vi "Patrick Builder.vi"() -> ()   [LabVIEW 2019, in "VIPM.lvclass"]
uses:
  VIPM.lvclass
  Typedefs/File Type--enum.ctl
  <vilib>/Utility/sysdir.llb/System Directory Type.ctl
  <vilib>/Utility/file.llb/Read Delimited Spreadsheet (string).vi
  <vilib>/Utility/file.llb/Write Delimited Spreadsheet (string).vi
  <vilib>/JKI/VIPM API/VIPM API_vipm_api.lvlib
panel:
  in  "Mode":T1
  in  "Create File List":bool
  out "Package Builder":string
  in  "Clear Notes":bool
  in  "Release Notes":string
  in  "Append Notes":bool
  in  "ALL":bool
  in  "Patch +1":bool
  out "Selected File List":string
  in  "Publish":bool
  in  "Open List":bool
  in  "Build":bool
  in  "Preview":bool
  out "Status":string
  in  "File List":i32(listbox)
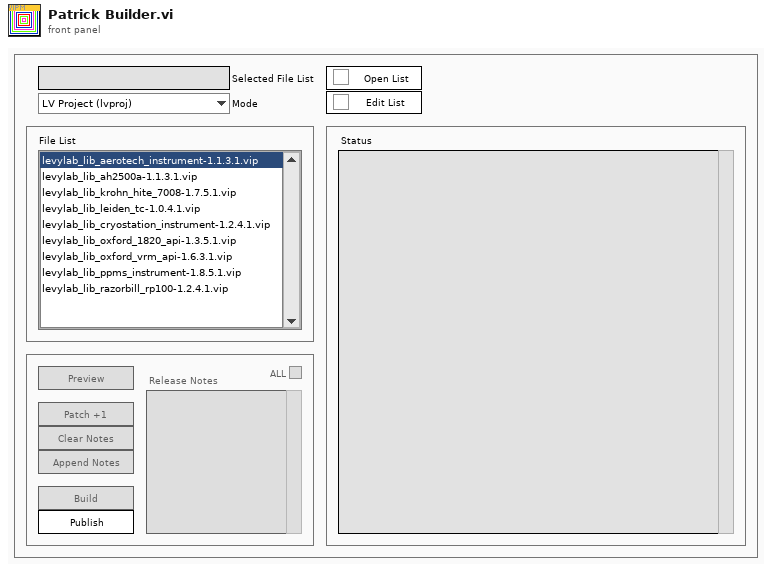
[diagram p1: front panel]
types:
  T1 = typedef "VIPM.lvclass/File Type--enum.ctl" = enum16{"LV Project (lvproj)", "Build Spec (vipb)", "Package (vip)"}
  T2 = enum32{"Invalid", "Standard", "Closed", "Hidden", "Minimized", "Maximized"}
  T3 = enum32{"invalid app kind", "Development System", "Run Time System", "Student Edition", "Embedded LabVIEW", "Evaluation", "Custom"}
  T4 = enum8{"Enabled", "Disabled", "Disabled and Grayed Out"}
  T5 = cluster{"Core":cluster{"Current VI Reference":refnum<vi>, "Close Panel on Exit?":bool}, "lvproj paths":path[], "vipb paths":path[], "vip paths":path[], "selected path":path, "config path":path, "Mode":T1}
  T6 = typedef "System Directory Type.ctl" = i32
  T7 = cluster{"Current VI Reference":refnum<vi>, "Close Panel on Exit?":bool}
  T8 = typedef "VIPM API_vipm_api.lvlib/VI Package Build Spec Data Cluster_vipm_api.ctl" = cluster{"Package Version":T9, "Product Name":string, "Company Name":string, "Author Name (Person or Company)":string, "Product Homepage (URL)":string, "Legal Copyright":string, "License Agreement Name":string, "Product Description Summary":string, "Product Description":string, "Release Notes - Change Log":string}
  T9 = typedef "VIPM API_vipm_api.lvlib/Version Info Cluster_vipm_api.ctl" = cluster{"major":u32, "minor":u32, "patch":u32, "build":u32}
  T10 = typedef "VIPM API_vipm_api.lvlib/Repository Info Cluster_vipm_api.ctl" = cluster{"Repository Name":string, "Repository Folder Location":path}
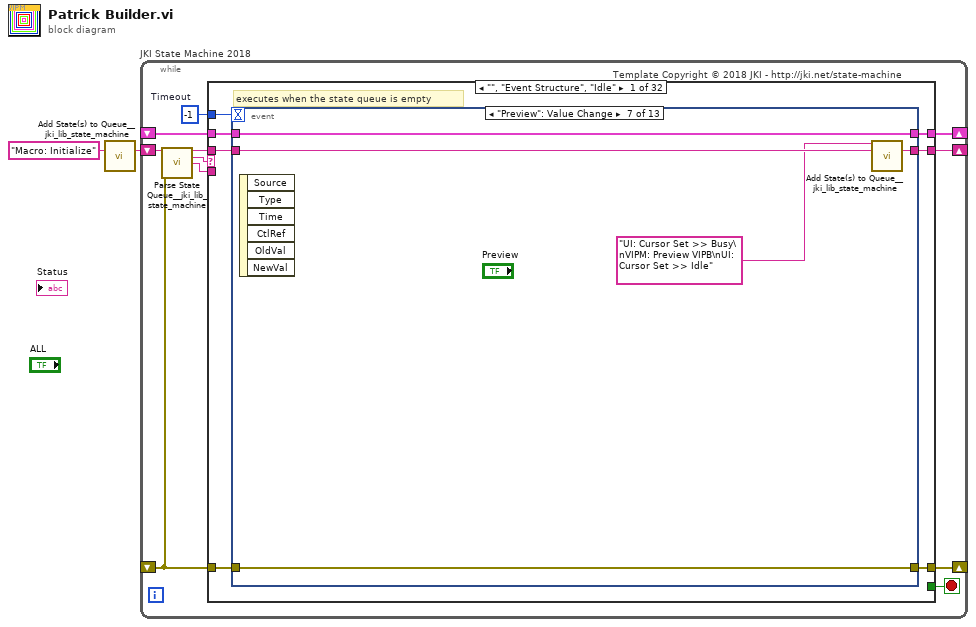
[diagram p0: block diagram]
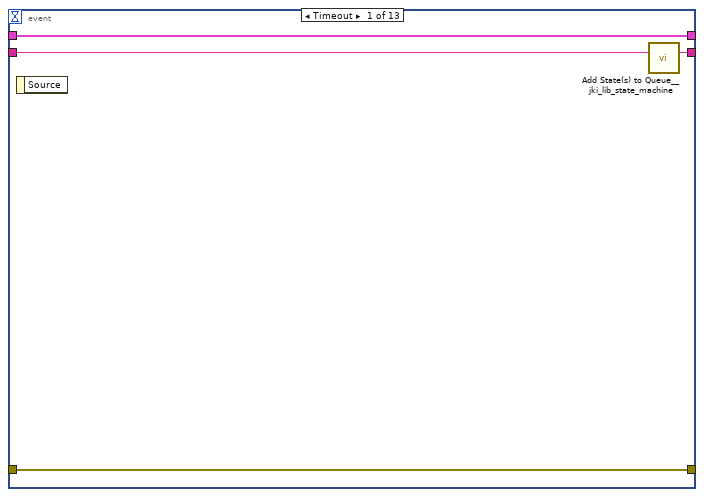
[diagram p2: hidden frame]
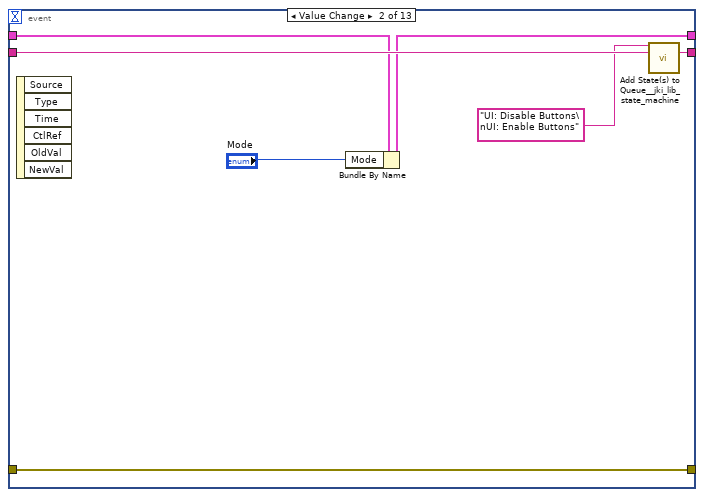
[diagram p3: hidden frame]
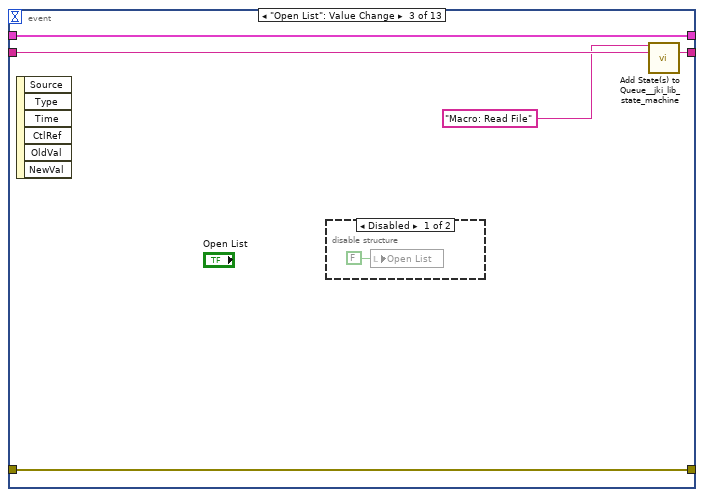
[diagram p4: hidden frame]
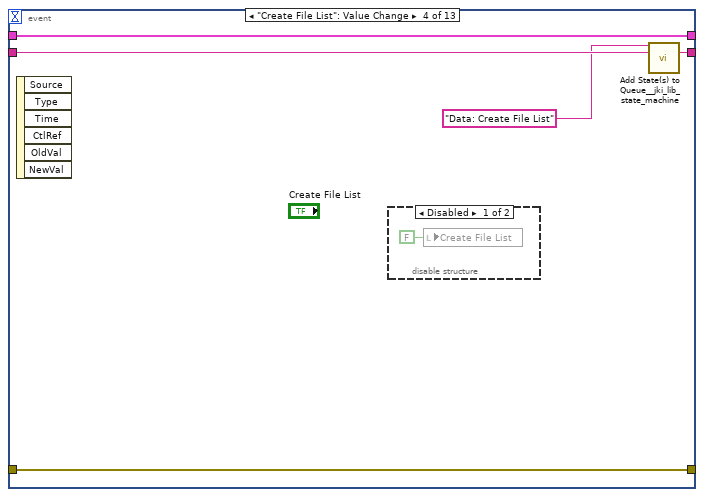
[diagram p6: hidden frame]
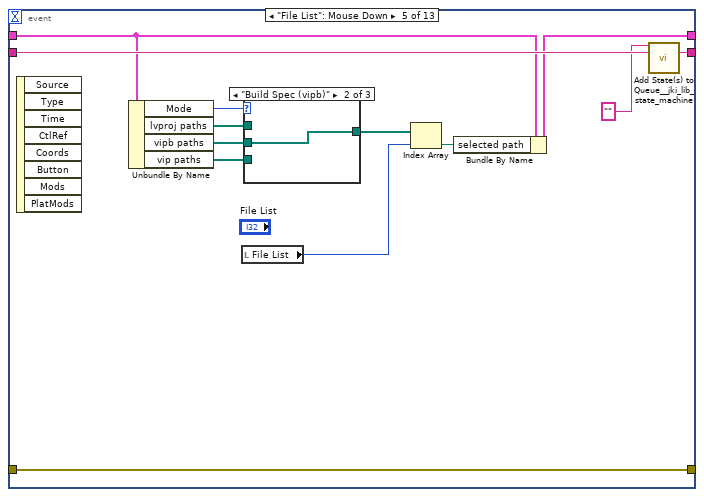
[diagram p8: hidden frame]
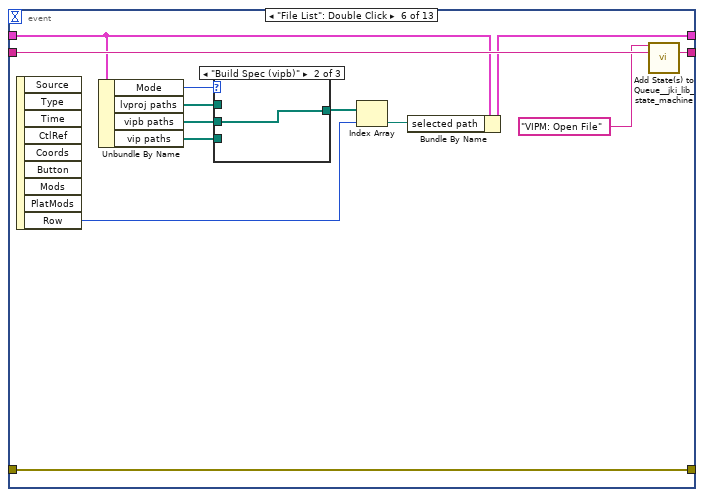
[diagram p11: hidden frame]
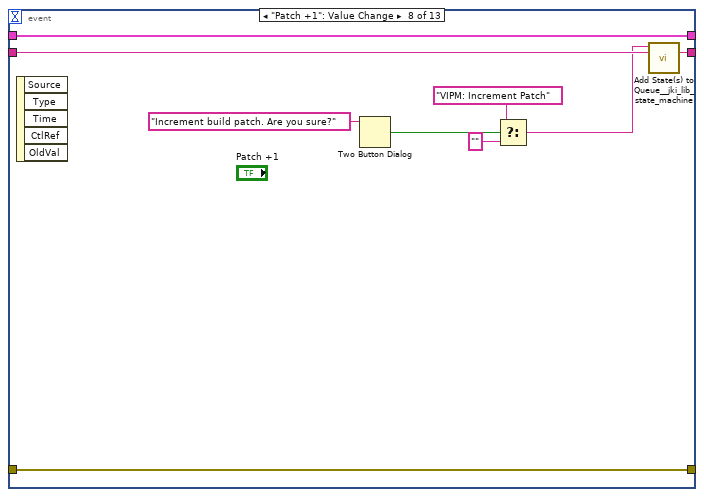
[diagram p14: hidden frame]
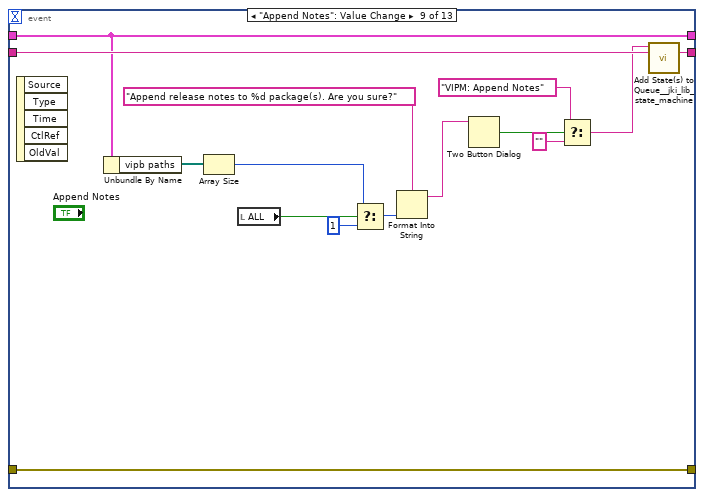
[diagram p15: hidden frame]
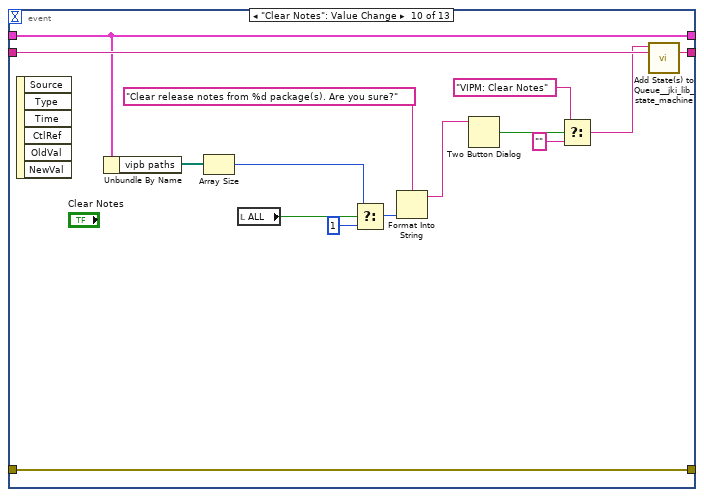
[diagram p16: hidden frame]
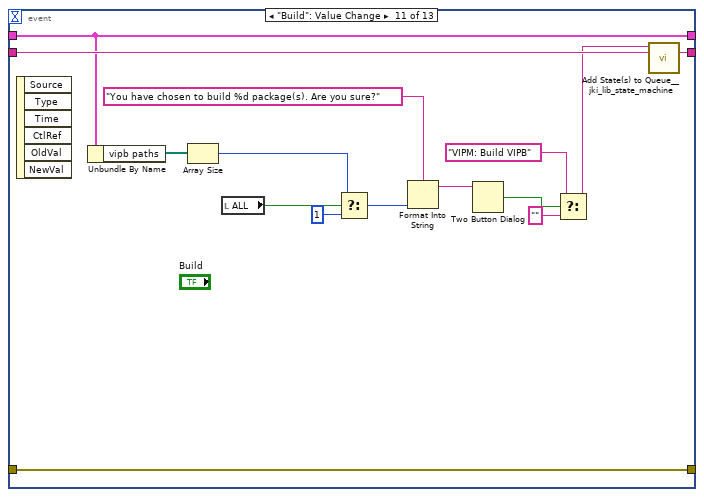
[diagram p17: hidden frame]
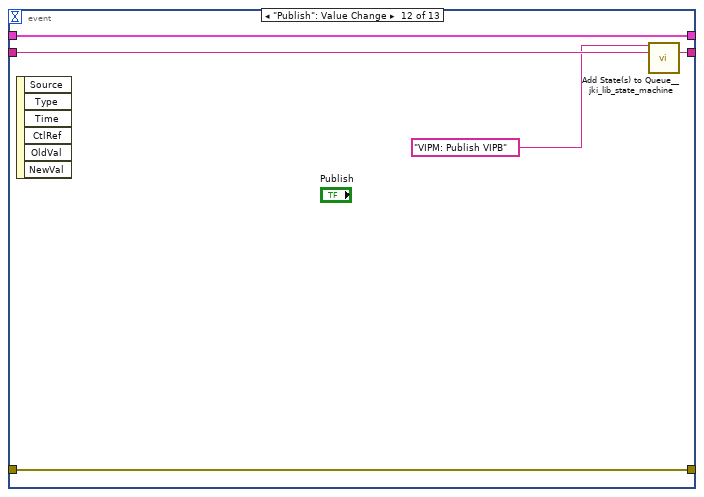
[diagram p18: hidden frame]
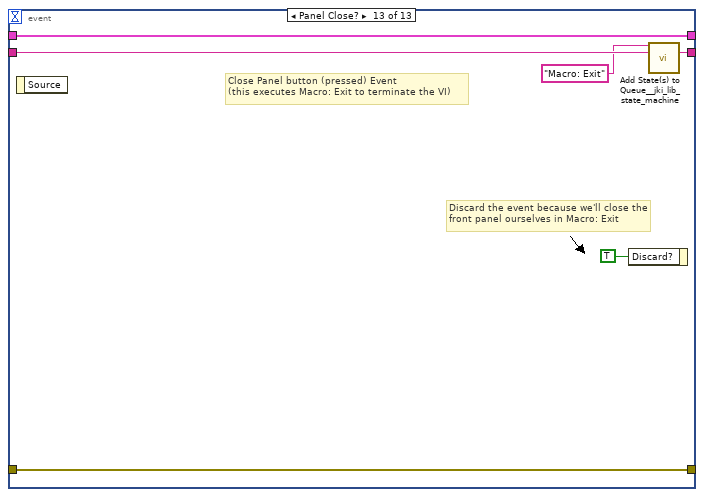
[diagram p19: hidden frame]
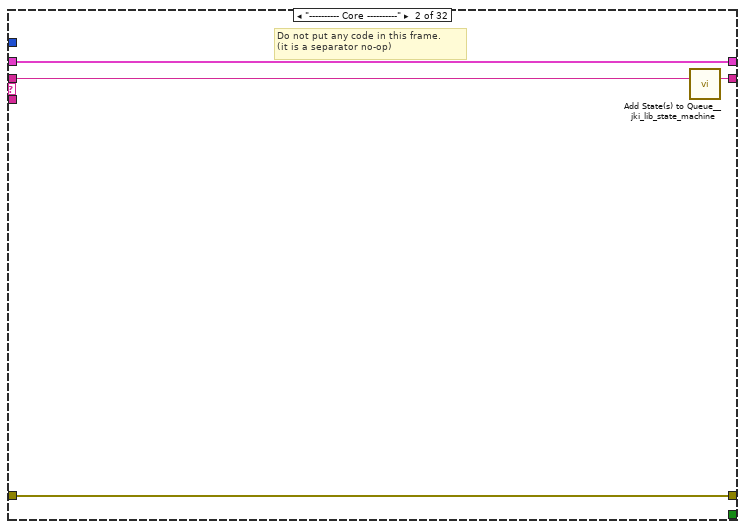
[diagram p20: hidden frame]
diagram:
  n1 = call <vilib>:"Add State(s) to Queue__jki_lib_state_machine.vi"("State(s) in (\"\")"="Macro: Initialize") -> ("States Out"=w2:string)  [unwired: 14 in]
  n2 = while "JKI State Machine 2018" {
    shift-right: [w6] -> _
    shift-left: _ -> [w5]
    shift-right: [w9] -> _
    shift-left: _ -> [w3]
    shift-right: [w8] -> _
    shift-left: w2 -> [w10]
    stop <- w7 stop-if-true
    w4 = -1  # Timeout
    # "Template Copyright © 2018 JKI - http://jki.net/state-machine"
    n3 = call <vilib>:"Parse State Queue__jki_lib_state_machine.vi"("State Queue"=w10, "Error In (no error)"=w3) -> ("Remaining States"=w12:string, "Current State"=w13:string, "Arguments"=w11:string)  [unwired: 11 in]
    n4 = case shown="\"\", \"Event Structure\", \"Idle\"" w13 {
      selector: w13 -> [_ _ w150 _ _ _ _ _ _ _ _ _ _ _ _ _ _ _ _ _ _ _ _ _ _ _ _ _ _ _ _ _]
      tunnel: w12 -> [w20 w149 w154 w173 w180 w189 w193 w213 w219 w229 w249 w266 w299 w332 w336 w346 w359 w377 w390 w401 w470 w475 w480 w490 w494 w507 w520 w540 w560 w579 w604 w625]
      tunnel: w11 -> [_ _ _ _ _ _ _ _ _ _ _ _ _ _ _ _ _ _ w385 w395 _ _ _ _ _ _ _ _ _ _ w592 _]
      tunnel: w5 -> [w18 w146 w152 w166 w177 w187 w190 _ w214 w221 w242 w258 w288 w330 w333 w344 w356 w372 w388 w397 w467 w472 w477 w487 w491 w505 w518 w538 w558 w577 w595 w619]
      tunnel: [w17 w147 w156 w170 errorcluster {"status"=FALSE, "code"=0, "source"=""} ("error out") w186 w191 w205 w215 w227 w239 w263 w289 w326 w334 w343 w357 w375 w386 w398 w468 w473 w478 w488 w492 w500 w509 w530 w549 w570 w598 w617] -> w9
      tunnel: w3 -> [w16 w147 w155 w170 w175 w186 w191 w204 w216 w227 w244 w264 w296 w327 w334 w342 w357 w375 w387 w399 w468 w473 w478 w488 w492 w499 w517 w533 w553 w572 w597 w616]
      tunnel: [w19 w148 w153 w172 w179 w188 w192 w212 w218 w228 w248 w265 w298 w331 w335 w345 w358 w376 w389 w400 w469 w474 w479 w489 w493 w506 w519 w539 w559 w578 w603 w624] -> w8
      tunnel: [_ _ _ _ _ TRUE _ _ _ _ _ _ _ _ _ _ _ _ _ _ _ _ _ _ _ _ _ _ _ _ _ _] -> w7
      tunnel: [w15 w146 w152 w171 w177 w187 w190 w211 w214 w225 w243 w262 w287 w330 w333 w344 w356 w372 w388 w397 w467 w472 w477 w487 w491 w505 w518 w538 w558 w577 w596 w619] -> w6
      tunnel: w4 -> [w14 _ _ _ _ _ _ _ _ _ _ _ _ _ _ _ _ _ _ _ _ _ _ _ _ _ _ _ _ _ _ _]
      frame "", "Event Structure", "Idle" {
        # "executes when the state queue is empty"
        n5 = event shown="[6] \"Preview\": Value Change" {
          selector: _ -> [_ _ _ _ _ _ _ _ _ _ _ _ _]
          dyn-events: _ -> [_ _ _ _ _ _ _ _ _ _ _ _ _]
          timeout: w14 -> [_ _ _ _ _ _ _ _ _ _ _ _ _]
          tunnel: w20 -> [w24 w31 w36 w42 w56 w72 w80 w89 w104 w119 w134 w139 w145]
          tunnel: [w23 w30 w35 w41 w55 w71 w79 w88 w103 w118 w133 w138 w144] -> w19
          tunnel: w18 -> [w21 w27 w32 w38 w53 w61 w77 w86 w90 w105 w126 w136 w142]
          tunnel: [w22 w29 w33 w39 w54 w70 w78 w87 w102 w117 w132 w137 w143] -> w17
          tunnel: w16 -> [w22 w29 w33 w39 w54 w70 w78 w87 w102 w117 w132 w137 w143]
          tunnel: [w21 w28 w32 w38 w52 w69 w77 w86 w90 w105 w126 w136 w142] -> w15
          event Timeout {
            n6 = event-data() -> ()  [unwired: 1 in, 1 out]
            n7 = call <vilib>:"Add State(s) to Queue__jki_lib_state_machine.vi"("State(s) in (\"\")"=w24) -> ("States Out"=w23:string)  [unwired: 14 in]
          }
          event Value Change {
            n8 = event-data() -> ()  [unwired: 1 in, 6 out]
            n9 = Bundle By Name(cluster=w27, "Mode"="Mode") -> (w28:T5)
            n10 = call <vilib>:"Add State(s) to Queue__jki_lib_state_machine.vi"("State(s) in Front (\"\")"="UI: Disable Buttons\nUI: Enable Buttons" ("State(s) in Front (\"\")"), "State(s) in (\"\")"=w31) -> ("States Out"=w30:string)  [unwired: 13 in]
          }
          event "Open List": Value Change {
            n11 = event-data() -> ()  [unwired: 1 in, 6 out]
            n12 = disable-structure shown="Disabled" {
              frame Disabled {
                n13 = local write "Open List"(FALSE ("Open List")) -> ()
              }
              frame Enabled {
              }
            }
            n14 = call <vilib>:"Add State(s) to Queue__jki_lib_state_machine.vi"("State(s) in Front (\"\")"="Macro: Read File" ("State(s) in Front (\"\")"), "State(s) in (\"\")"=w36) -> ("States Out"=w35:string)  [unwired: 13 in]
          }
          event "Create File List": Value Change {
            n15 = event-data() -> ()  [unwired: 1 in, 6 out]
            n16 = disable-structure shown="Disabled" {
              frame Disabled {
                n17 = local write "Create File List"(FALSE ("Create File List")) -> ()
              }
              frame Enabled {
              }
            }
            n18 = call <vilib>:"Add State(s) to Queue__jki_lib_state_machine.vi"("State(s) in Front (\"\")"="Data: Create File List" ("State(s) in Front (\"\")"), "State(s) in (\"\")"=w42) -> ("States Out"=w41:string)  [unwired: 13 in]
          }
          event "File List": Mouse Down {
            n19 = event-data() -> ()  [unwired: 1 in, 8 out]
            n20 = Unbundle By Name(w53) -> ("Mode"=w48:T1, "lvproj paths"=w45:path[], "vipb paths"=w44:path[], "vip paths"=w46:path[])
            n21 = local read "File List"() -> (w49:i32)
            n22 = case shown="\"Build Spec (vipb)\"" w48 {
              tunnel: [w57 w58 w59] -> w47
              tunnel: w46 -> [_ _ w59]
              tunnel: w45 -> [w57 _ _]
              tunnel: w44 -> [_ w58 _]
              frame "LV Project (lvproj)", Default {
              }
              frame "Build Spec (vipb)" {
              }
              frame "Package (vip)" {
              }
            }
            n23 = Index Array(array=w47, index=w49) -> (element=w51:path)
            n24 = Bundle By Name(cluster=w53, "selected path"=w51) -> (w52:T5)
            n25 = call <vilib>:"Add State(s) to Queue__jki_lib_state_machine.vi"("State(s) in Front (\"\")"="" ("State(s) in Front (\"\")"), "State(s) in (\"\")"=w56) -> ("States Out"=w55:string)  [unwired: 13 in]
          }
          event "File List": Double Click {
            n26 = event-data() -> ("Row"=w66:i32)  [unwired: 1 in, 8 out]
            n27 = Unbundle By Name(w61) -> ("Mode"=w65:T1, "lvproj paths"=w63:path[], "vipb paths"=w62:path[], "vip paths"=w64:path[])
            n28 = case shown="\"Build Spec (vipb)\"" w65 {
              tunnel: [w73 w74 w75] -> w60
              tunnel: w64 -> [_ _ w75]
              tunnel: w63 -> [w73 _ _]
              tunnel: w62 -> [_ w74 _]
              frame "LV Project (lvproj)", Default {
              }
              frame "Build Spec (vipb)" {
              }
              frame "Package (vip)" {
              }
            }
            n29 = Index Array(array=w60, index=w66) -> (element=w68:path)
            n30 = Bundle By Name(cluster=w61, "selected path"=w68) -> (w69:T5)
            n31 = call <vilib>:"Add State(s) to Queue__jki_lib_state_machine.vi"("State(s) in Front (\"\")"="VIPM: Open File" ("State(s) in Front (\"\")"), "State(s) in (\"\")"=w72) -> ("States Out"=w71:string)  [unwired: 13 in]
          }
          event "Preview": Value Change {
            n32 = event-data() -> ()  [unwired: 1 in, 6 out]
            n33 = call <vilib>:"Add State(s) to Queue__jki_lib_state_machine.vi"("State(s) in Front (\"\")"="UI: Cursor Set >> Busy\nVIPM: Preview VIPB\nUI: Cursor Set >> Idle" ("State(s) in Front (\"\")"), "State(s) in (\"\")"=w80) -> ("States Out"=w79:string)  [unwired: 13 in]
          }
          event "Patch +1": Value Change {
            n34 = event-data() -> ()  [unwired: 1 in, 5 out]
            n35 = Two Button Dialog(message="Increment build patch. Are you sure?") -> (T button?=w84:bool)  [unwired: 2 in]
            n36 = Select(t="VIPM: Increment Patch" ("State(s) in Front (\"\")"), s=w84, f="") -> (s? t:f=w81:string)
            n37 = call <vilib>:"Add State(s) to Queue__jki_lib_state_machine.vi"("State(s) in Front (\"\")"=w81, "State(s) in (\"\")"=w89) -> ("States Out"=w88:string)  [unwired: 13 in]
          }
          event "Append Notes": Value Change {
            n38 = event-data() -> ()  [unwired: 1 in, 5 out]
            n39 = Unbundle By Name(w90) -> ("vipb paths"=w97:path[])
            n40 = Array Size(array=w97) -> (size(s)=w95:i32)
            n41 = local read "ALL"() -> (w96:bool)
            n42 = Select(t=w95, s=w96, f=1) -> (s? t:f=w98:i32)
            n43 = Format Into String(format string="Append release notes to %d package(s). Are you sure?" ("message"), w98) -> (resulting string=w92:string)  [unwired: 2 in, 1 out]
            n44 = Two Button Dialog(message=w92) -> (T button?=w101:bool)  [unwired: 2 in]
            n45 = Select(t="VIPM: Append Notes" ("State(s) in Front (\"\")"), s=w101, f="") -> (s? t:f=w99:string)
            n46 = call <vilib>:"Add State(s) to Queue__jki_lib_state_machine.vi"("State(s) in Front (\"\")"=w99, "State(s) in (\"\")"=w104) -> ("States Out"=w103:string)  [unwired: 13 in]
          }
          event "Clear Notes": Value Change {
            n47 = event-data() -> ()  [unwired: 1 in, 6 out]
            n48 = Unbundle By Name(w105) -> ("vipb paths"=w112:path[])
            n49 = Array Size(array=w112) -> (size(s)=w110:i32)
            n50 = local read "ALL"() -> (w111:bool)
            n51 = Select(t=w110, s=w111, f=1) -> (s? t:f=w113:i32)
            n52 = Format Into String(format string="Clear release notes from %d package(s). Are you sure?" ("message"), w113) -> (resulting string=w107:string)  [unwired: 2 in, 1 out]
            n53 = Two Button Dialog(message=w107) -> (T button?=w116:bool)  [unwired: 2 in]
            n54 = Select(t="VIPM: Clear Notes" ("State(s) in Front (\"\")"), s=w116, f="") -> (s? t:f=w114:string)
            n55 = call <vilib>:"Add State(s) to Queue__jki_lib_state_machine.vi"("State(s) in Front (\"\")"=w114, "State(s) in (\"\")"=w119) -> ("States Out"=w118:string)  [unwired: 13 in]
          }
          event "Build": Value Change {
            n56 = event-data() -> ()  [unwired: 1 in, 6 out]
            n57 = Unbundle By Name(w126) -> ("vipb paths"=w125:path[])
            n58 = Array Size(array=w125) -> (size(s)=w123:i32)
            n59 = local read "ALL"() -> (w124:bool)
            n60 = Select(t=w123, s=w124, f=1) -> (s? t:f=w121:i32)
            n61 = Format Into String(format string="You have chosen to build %d package(s). Are you sure?" ("message"), w121) -> (resulting string=w120:string)  [unwired: 2 in, 1 out]
            n62 = Two Button Dialog(message=w120) -> (T button?=w130:bool)  [unwired: 2 in]
            n63 = Select(t="VIPM: Build VIPB" ("State(s) in Front (\"\")"), s=w130, f="") -> (s? t:f=w127:string)
            n64 = call <vilib>:"Add State(s) to Queue__jki_lib_state_machine.vi"("State(s) in Front (\"\")"=w127, "State(s) in (\"\")"=w134) -> ("States Out"=w133:string)  [unwired: 13 in]
          }
          event "Publish": Value Change {
            n65 = event-data() -> ()  [unwired: 1 in, 6 out]
            n66 = call <vilib>:"Add State(s) to Queue__jki_lib_state_machine.vi"("State(s) in Front (\"\")"="VIPM: Publish VIPB" ("State(s) in Front (\"\")"), "State(s) in (\"\")"=w139) -> ("States Out"=w138:string)  [unwired: 13 in]
          }
          event Panel Close? {
            # "Discard the event because we'll close the front panel ourselves in Macro: Exit"
            # "Close Panel button (pressed) Event\n(this executes Macro: Exit to terminate the VI)"
            n67 = event-data() -> ()  [unwired: 1 in, 1 out]
            n68 = event-data("Discard?"=TRUE) -> ()  [unwired: 1 in, 1 out]
            n69 = call <vilib>:"Add State(s) to Queue__jki_lib_state_machine.vi"("State(s) in Front (\"\")"="Macro: Exit", "State(s) in (\"\")"=w145) -> ("States Out"=w144:string)  [unwired: 13 in]
          }
        }
      }
      frame "---------- Core ----------" {
        # "Do not put any code in this frame.\n(it is a separator no-op)"
        n70 = call <vilib>:"Add State(s) to Queue__jki_lib_state_machine.vi"("State(s) in (\"\")"=w149) -> ("States Out"=w148:string)  [unwired: 14 in]
      }
      frame Default {
        w159 = 42 items=["No error", "Argument error", "Memory is full", "Out of zone", "End of file", "File already open", "Generic file I/O error", "File not found", "File permission error", "Disk is full", "Duplicate path", "Too many files open", "System feature not enabled", "Resource file not found", "Cannot add resource", "Resource not found", "Image not found", "Image memory error", "Pen does not exist", "Config type invalid", "Config token not found", "Config parse error", "Config memory error", "Bad external code format", "Bad external code offset", "External code not present", "Null window", "Destroy window error", "Null menu", "Print aborted", "Bad print record", "Print driver error", "Windows error during printing", "Memory error during printing", "Print dialog error", "Generic print error", "Invalid device refnum", "Device not found", "Device parameter error", "Device unit error", "Cannot open device", "Device call aborted", "Generic error", "Cancelled by user", "Object ID too low", "Object ID too high", "Object not in heap", "Unknown heap", "Unknown object (invalid DefProc)", "Unknown object (DefProc not in table)", "Message out of range", "Invalid (null) method", "Unknown message", "Manager call not supported", "Bad address", "Network operation in progress", "Network operation timed out", "Connection is busy", "Network attribute not supported", "Network error", "Address in use", "System out of memory", "Connection aborted", "Connection refused", "Not connected", "Already connected", "Connection closed", "Initialization error (interapplication manager)", "Bad occurrence", "Wait on unbound occurrence handler", "Occurrence queue overflow", "Datalog type conflict", "Unused", "Unrecognized type (interapplication manager)", "Memory corrupt", "Failed to make temporary DLL", "Old CIN version", "Drag socket not found", "Failed to load drop-object", "Failed to register OLE object", "Failed to release OLE object", "Format specifier type mismatch", "Unknown format specifier", "Too few format specifiers", "Too many format specifiers", "Scan failed", "Newer CIN version", "Error converting to variant", "Runtime menu error", "Password tampered", "Variant attribute not found", "Incompatible variant data type", "Event data is not available", "Event Store is not present", "Occurrence is not found", "Event Queue is not created", "Event info is not available", "Refnum passed is NULL", "Error retrieving Class GUID", "Error retrieving CoClass GUID", "Error retrieving TypeLib GUID.", "Bad built application magic bytes.", "Specific driver is different from the specific driver associated with the Logical Name.", "There is no session opened to the class driver.", "Max Error", "MAX - Error with config objects", "MAX - Error loading configuration", "MAX - Group not supported"]
        # "Current State"
        # "Do not delete, rename, or modify this frame.\n(this is used to capture unhandled states and typos)"
        # "Handle mistyped state name (developer tool)"
        n71 = Format Into String(format string="Software Exception: Unhandled State \"%s\"." ("message"), error in=w155, w150) -> (resulting string=w158:string, error out=w157:errorcluster)  [unwired: 1 in]
        n72 = call <vilib>:"Error Cluster From Error Code.vi"("show call chain? (False)"=TRUE, "error in (no error)"=w157, "error message (\"\")"=w158, "error code (0)"=w159) -> ("error out"=w156:errorcluster)  [unwired: 5 in]
        n73 = call <vilib>:"Add State(s) to Queue__jki_lib_state_machine.vi"("State(s) in (\"\")"=w154) -> ("States Out"=w153:string)  [unwired: 14 in]
      }
      frame "Initialize Core Data" {
        # "Do not delete, rename, or modify this frame.\n(this is used to determine panel behavior on exit)"
        # "originally closed?"
        # "exe?"
        # "If panel starts closed or is an EXE, then close it when we exit"
        n74 = property class="VI"() -> ("FP.State"=w163:T2)  [unwired: 2 in, 2 out]
        n75 = property class="App"() -> ("App.Kind"=w169:T3)  [unwired: 2 in, 2 out]
        n76 = control-ref of="Current VI Reference"() -> (w164:refnum<vi>)
        n77 = Equal?(x=w163, y=T2."Closed" ("Front Panel Window:State")) -> (x = y?=w161:bool)
        n78 = Equal?(x=w169, y=T3."Run Time System" ("Application:Kind")) -> (x = y?=w167:bool)
        n79 = Or(x=w161, y=w167) -> (x .or. y?=w165:bool)
        n80 = Bundle By Name(cluster=w166, "Core.Current VI Reference"=w164, "Core.Close Panel on Exit?"=w165) -> (w171:T5)
        n81 = call <vilib>:"Add State(s) to Queue__jki_lib_state_machine.vi"("State(s) in (\"\")"=w173) -> ("States Out"=w172:string)  [unwired: 14 in]
      }
      frame "Error Handler" {
        # "Unhandled Error -- Display it"
        # "Handle any errors here.\nYou can also output any states to clean-up after errors occur"
        # "Clear error"
        n82 = case shown="Error 1059" w175 {
          selector: w175 -> [w181 w182 _]
          tunnel: [w181 w182 w183] -> w174
          frame No Error {
          }
          frame Default {
          }
          frame Error {
            n83 = property on="Open List" class="Bool"("Val(Sgnl)"=TRUE) -> (error out=w183:errorcluster)  [unwired: 2 in, 1 out]
          }
        }
        n84 = call <vilib>:"General Error Handler.vi"("error in (no error)"=w174) -> ()  [unwired: 10 in, 5 out]
        n85 = call <vilib>:"Add State(s) to Queue__jki_lib_state_machine.vi"("State(s) in Front (\"\")"="/* Post Error States", "State(s) in (\"\")"=w180) -> ("States Out"=w179:string)  [unwired: 13 in]
      }
      frame "Exit" {
        # "Do not put any code in this frame.\n(No errors that occur here will be handled.)"
        n86 = call <vilib>:"Add State(s) to Queue__jki_lib_state_machine.vi"("State(s) in (\"\")"=w189) -> ("States Out"=w188:string)  [unwired: 14 in]
      }
      frame "---------- Data ----------" {
        # "Do not put any code in this frame.\n(It is a separator no-op. You can make a copy of this frame to create a new Data frame)"
        n87 = call <vilib>:"Add State(s) to Queue__jki_lib_state_machine.vi"("State(s) in (\"\")"=w193) -> ("States Out"=w192:string)  [unwired: 14 in]
      }
      frame "Data: Initialize" {
        w194 = File_Type--enum."LV Project (lvproj)"  # Mode
        w200 = T6 3 items=["User Home"=0, "User Desktop"=1, "User Documents"=2, "User Application Data"=3, "User Preferences"=4, "User Temporary"=5, "Public Documents"=6, "Public Application Data"=7, "Public Preferences"=8, "Public Cache"=13, "System Core Libraries"=9, "System Installed Libraries"=10, "Application Files"=11, "Boot Volume Root"=12] ("system directory type")
        w201 = path[] []  # lvproj paths
        w202 = path[] []  # vip paths
        w203 = path[] []  # vipb paths
        w207 = path ""  # config path
        w209 = path ""  # selected path
        w210 = T7 {"Current VI Reference"=refnum, "Close Panel on Exit?"=FALSE}  # Core
        # "Initialize the shift-register data, here.\n(data names are defined by what you wire into the bundle function)"
        n88 = call <vilib>:"Get System Directory.vi"("system directory type"=w200) -> ("system directory"=w197:path)  [unwired: 10 in]
        n89 = Build Path(base path=w197, name or relative path="LevyLab") -> (appended path=w196:path)
        n90 = Build Path(base path=w196, name or relative path="build-support") -> (appended path=w198:path)
        n91 = call <userlib>:"Create Dir if Non-Existant__ogtk.vi"("error in (no error)"=w204, "Directory Path"=w198) -> ("error out"=w205:errorcluster, "dup Directory Path"=w206:path)  [unwired: 7 in, 1 out]
        n92 = Variant To Data(type=w207, Variant=w206) -> (data=w208:path)  [unwired: 1 in, 1 out]
        n93 = Bundle("Core"=w210, "lvproj paths"=w201, "vipb paths"=w203, "vip paths"=w202, "selected path"=w209, "config path"=w208, "Mode"=w194) -> (w211:T5)  [unwired: 1 in]
        n94 = call <vilib>:"Add State(s) to Queue__jki_lib_state_machine.vi"("State(s) in (\"\")"=w213) -> ("States Out"=w212:string)  [unwired: 14 in]
      }
      frame "Data: Cleanup" {
        # "Cleanup any data and references, here.\n(this is called automatically, by the Macro: Exit)"
        n95 = Unbundle By Name(w214) -> ("Core.Current VI Reference"=w217:refnum<vi>)
        n96 = Close Reference(reference=w217, error in (no error)=w216) -> (error out=w215:errorcluster)
        n97 = call <vilib>:"Add State(s) to Queue__jki_lib_state_machine.vi"("State(s) in (\"\")"=w219) -> ("States Out"=w218:string)  [unwired: 14 in]
      }
      frame "Data: Update Listbox" {
        w223 = 0 ("Value (Signaling)")
        # "Do not put any code in this frame.\n(It is a separator no-op. You can make a copy of this frame to create a new Data frame)"
        n98 = Unbundle By Name(w221) -> ("Mode"=w222:T1)
        n99 = case shown="\"Package (vip)\"" w222 {
          tunnel: w221 -> [w231 w233 w235]
          tunnel: [w230 w232 w234] -> w220
          frame "LV Project (lvproj)", Default {
            n100 = Unbundle By Name(w231) -> ("lvproj paths"=w230:path[])
          }
          frame "Build Spec (vipb)" {
            n101 = Unbundle By Name(w233) -> ("vipb paths"=w232:path[])
          }
          frame "Package (vip)" {
            n102 = Unbundle By Name(w235) -> ("vip paths"=w234:path[])
          }
        }
        n103 = for {
          tunnel: w220 -> [w237] mode=indexing
          tunnel: [w236] -> w226 mode=indexing
          n104 = Strip Path(path=w237) -> (name=w236:string)  [unwired: 1 out]
        }
        n105 = property on="File List" class="LstBox (strict)"("Item Names"=w226, "Val(Sgnl)"=w223) -> ()  [unwired: 2 in, 2 out]
        n106 = Index Array(array=w220, index=w223) -> (element=w224:path)
        n107 = Bundle By Name(cluster=w221, "selected path"=w224) -> (w225:T5)
        n108 = call <vilib>:"Add State(s) to Queue__jki_lib_state_machine.vi"("State(s) in (\"\")"=w229) -> ("States Out"=w228:string)  [unwired: 14 in]
      }
      frame "Data: Choose File List" {
        # "Do not put any code in this frame.\n(It is a separator no-op. You can make a copy of this frame to create a new Data frame)"
        n109 = Unbundle By Name(w242) -> ("config path"=w247:path)
        n110 = call "File Dialog"("start path"=w247, "error in"=w244, "pattern (all files)"="*.txt") -> ("selected path"=w246:path, "cancelled"=w241:bool, "error out"=w240:errorcluster)  [unwired: 9 in, 1 out]
        n111 = case shown="False" w241 {
          tunnel: w246 -> [w250 _]
          tunnel: [w254 _] -> w245
          tunnel: [w253 w255] -> w243
          tunnel: w242 -> [w252 w255]
          tunnel: w240 -> [w251 _]
          tunnel: [w251 _] -> w239
          frame False {
            n112 = Bundle By Name(cluster=w252, "config path"=w250) -> (w253:T5)
            n113 = Strip Path(path=w250) -> (name=w254:string)  [unwired: 1 out]
          }
          frame True {
          }
        }
        "Selected File List" <- w245
        n114 = call <vilib>:"Add State(s) to Queue__jki_lib_state_machine.vi"("State(s) in (\"\")"=w249) -> ("States Out"=w248:string)  [unwired: 14 in]
      }
      frame "Data: Create File List" {
        # "Do not put any code in this frame.\n(It is a separator no-op. You can make a copy of this frame to create a new Data frame)"
        n115 = Unbundle By Name(w258) -> ("config path"=w257:path, "Mode"=w256:T1)
        n116 = call "Build File List Window.vi"("error in"=w264, "File Type"=w256, "Path"=w257) -> ("error out"=w263:errorcluster, "File Type out"=w261:T1, "files out"=w260:path[])  [unwired: 6 in]
        n117 = Empty Array?(array=w260) -> (empty?=w259:bool)
        n118 = case shown="False" w259 {
          tunnel: [w270 w283] -> w262
          tunnel: w258 -> [w269 w283]
          tunnel: w261 -> [w268 _]
          tunnel: w260 -> [w267 _]
          frame False {
            n119 = case shown="\"Package (vip)\"" w268 {
              selector: w268 -> [w271 w275 w279]
              tunnel: [w274 w278 w282] -> w270
              tunnel: w269 -> [w273 w277 w281]
              tunnel: w267 -> [w272 w276 w280]
              frame "LV Project (lvproj)" {
                n120 = Bundle By Name(cluster=w273, "lvproj paths"=w272, "Mode"=w271) -> (w274:T5)
              }
              frame "Build Spec (vipb)" {
                n121 = Bundle By Name(cluster=w277, "vipb paths"=w276, "Mode"=w275) -> (w278:T5)
              }
              frame "Package (vip)" {
                n122 = Bundle By Name(cluster=w281, "vip paths"=w280, "Mode"=w279) -> (w282:T5)
              }
            }
          }
          frame True {
          }
        }
        n123 = call <vilib>:"Add State(s) to Queue__jki_lib_state_machine.vi"("State(s) in (\"\")"=w266) -> ("States Out"=w265:string)  [unwired: 14 in]
      }
      frame "Data: Read File List" {
        # "Do not put any code in this frame.\n(It is a separator no-op. You can make a copy of this frame to create a new Data frame)"
        n124 = Unbundle By Name(w288) -> ("config path"=w297:path)
        n125 = call-poly <vilib>:"Read Delimited Spreadsheet.vi"("file path (dialog if empty)"=w297, "error in (no error)"=w296, "transpose? (F)"=TRUE, "delimiter (\\t)"="\\n" ("delimiter (\\t)")) -> ("all rows"=w294:string[][], "error out"=w290:errorcluster)  [unwired: 6 in, 4 out]
        n126 = Index Array(array=w294) -> (element=w293:string[])  [unwired: 2 in]
        n127 = String To Path(string=w293) -> (path=w291:path[])
        n128 = for {
          tunnel: w291 -> [w322] mode=indexing
          tunnel: w290 -> [w321]
          tunnel: [w320] -> w289
          tunnel: [w318] -> w286 mode=indexing
          tunnel: [w317] -> w284
          n129 = call <vilib>:"Get File Extension.vi"("error in (no error)"=w321, "file"=w322) -> ("error out"=w320:errorcluster, "lowercase file extension"=w319:string, "dup file"=w318:path)  [unwired: 5 in, 2 out]
          n130 = call "Extension to Mode.vi"("lowercase file extension"=w319) -> ("Mode"=w317:T1)  [unwired: 10 in]
        }
        n131 = Empty Array?(array=w286) -> (empty?=w285:bool)
        n132 = case shown="False" w285 {
          tunnel: [w303 w316] -> w287
          tunnel: w288 -> [w302 w316]
          tunnel: w284 -> [w300 _]
          tunnel: w286 -> [w301 _]
          frame False {
            n133 = case shown="\"Build Spec (vipb)\"" w300 {
              selector: w300 -> [w304 w308 w312]
              tunnel: [w307 w311 w315] -> w303
              tunnel: w302 -> [w306 w310 w314]
              tunnel: w301 -> [w305 w309 w313]
              frame "LV Project (lvproj)" {
                n134 = Bundle By Name(cluster=w306, "lvproj paths"=w305, "Mode"=w304) -> (w307:T5)
              }
              frame "Build Spec (vipb)" {
                n135 = Bundle By Name(cluster=w310, "vipb paths"=w309, "Mode"=w308) -> (w311:T5)
              }
              frame "Package (vip)" {
                n136 = Bundle By Name(cluster=w314, "vip paths"=w313, "Mode"=w312) -> (w315:T5)
              }
            }
            n137 = local write "Mode"(w300) -> ()
          }
          frame True {
          }
        }
        n138 = call <vilib>:"Add State(s) to Queue__jki_lib_state_machine.vi"("State(s) in (\"\")"=w299) -> ("States Out"=w298:string)  [unwired: 14 in]
      }
      frame "Data: Save File List" {
        # "Do not put any code in this frame.\n(It is a separator no-op. You can make a copy of this frame to create a new Data frame)"
        n139 = Unbundle By Name(w330) -> ("config path"=w325:path, "vipb paths"=w329:path[])
        n140 = Path To String(path=w329) -> (string=w328:string[])
        n141 = call-poly <vilib>:"Write Delimited Spreadsheet.vi"("file path (dialog if empty)"=w325, "1D data"=w328, "error in (no error)"=w327, "transpose? (no:F)"=TRUE, "delimiter (\\t)"="\\n" ("delimiter (\\t)")) -> ("error out"=w326:errorcluster)  [unwired: 9 in, 1 out]
        n142 = call <vilib>:"Add State(s) to Queue__jki_lib_state_machine.vi"("State(s) in (\"\")"=w332) -> ("States Out"=w331:string)  [unwired: 14 in]
      }
      frame "---------- UI ----------" {
        # "Do not put any code in this frame.\n(It is a separator no-op. You can make a copy of this frame to create a new UI frame)"
        n143 = call <vilib>:"Add State(s) to Queue__jki_lib_state_machine.vi"("State(s) in (\"\")"=w336) -> ("States Out"=w335:string)  [unwired: 14 in]
      }
      frame "UI: Initialize" {
        # "Initialize the User Interface, here.\n(this is called automatically, by the Macro: Init)"
        n144 = call <userlib>:"MGI Get Executable Version.vi"() -> ("Version"=w339:string)  [unwired: 7 in]
        n145 = local write "Status"("" ("Status")) -> ()
        n146 = Format Into String(format string="Patrick Builder v%s", w339) -> (resulting string=→"Package Builder":string)  [unwired: 2 in, 1 out]
        n147 = call <userlib>:"Fit VI window to Largest Dec__ogtk.vi"("error in (no error)"=w342, "border spacing (2 px)"=0) -> ("error out"=w343:errorcluster)  [unwired: 4 in, 1 out]
        n148 = call <vilib>:"Add State(s) to Queue__jki_lib_state_machine.vi"("State(s) in (\"\")"=w346) -> ("States Out"=w345:string)  [unwired: 14 in]
      }
      frame "UI: Disable Buttons" {
        # "Do not put any code in this frame.\n(It is a separator no-op. You can make a copy of this frame to create a new UI frame)"
        n149 = control-ref of="Preview"() -> (w355:refnum<vi>)
        n150 = control-ref of="Build"() -> (w354:refnum<vi>)
        n151 = control-ref of="Publish"() -> (w352:refnum<vi>)
        n152 = control-ref of="Clear Notes"() -> (w351:refnum<vi>)
        n153 = control-ref of="Append Notes"() -> (w350:refnum<vi>)
        n154 = control-ref of="Patch +1"() -> (w349:refnum<vi>)
        n155 = control-ref of="Release Notes"() -> (w348:refnum<vi>)
        n156 = control-ref of="ALL"() -> (w347:refnum<vi>)
        n157 = Build Array(w355, w354, w352, w351, w350, w349, w348, w347) -> (w353:refnum<vi>[])
        n158 = for {
          tunnel: w353 -> [w360] mode=indexing
          n159 = property class="Ctl"(reference=w360, "DisabledEnum"=T4."Disabled and Grayed Out" ("Disabled")) -> ()  [unwired: 1 in, 2 out]
        }
        n160 = call <vilib>:"Add State(s) to Queue__jki_lib_state_machine.vi"("State(s) in (\"\")"=w359) -> ("States Out"=w358:string)  [unwired: 14 in]
      }
      frame "UI: Enable Buttons" {
        # "Do not put any code in this frame.\n(It is a separator no-op. You can make a copy of this frame to create a new UI frame)"
        n161 = Unbundle By Name(w372) -> ("Mode"=w364:T1, "vipb paths"=w362:path[])
        n162 = control-ref of="Preview"() -> (w374:refnum<vi>)
        n163 = control-ref of="Build"() -> (w373:refnum<vi>)
        n164 = control-ref of="Clear Notes"() -> (w371:refnum<vi>)
        n165 = control-ref of="Append Notes"() -> (w370:refnum<vi>)
        n166 = control-ref of="Patch +1"() -> (w368:refnum<vi>)
        n167 = control-ref of="Release Notes"() -> (w367:refnum<vi>)
        n168 = control-ref of="ALL"() -> (w366:refnum<vi>)
        n169 = Empty Array?(array=w362) -> (empty?=w365:bool)
        n170 = Build Array(w374, w373, w371, w370, w368, w367, w366) -> (w369:refnum<vi>[])
        n171 = Not(x=w365) -> (.not. x?=w363:bool)
        n172 = case shown="\"LV Project (lvproj)\"" w364 {
          tunnel: w369 -> [_ _ w381]
          tunnel: w363 -> [_ _ w380]
          frame "Package (vip)" {
            n173 = control-ref of="Publish"() -> (w378:refnum<vi>)
            n174 = property class="Bool"(reference=w378, "DisabledEnum"=T4."Enabled" ("Disabled")) -> ()  [unwired: 1 in, 2 out]
          }
          frame "LV Project (lvproj)" {
          }
          frame "Build Spec (vipb)" {
            n175 = case shown="True" w380 {
              tunnel: w381 -> [_ w382]
              frame False {
              }
              frame True {
                n176 = for {
                  tunnel: w382 -> [w383] mode=indexing
                  n177 = property class="Ctl"(reference=w383, "DisabledEnum"=T4."Enabled" ("Disabled")) -> ()  [unwired: 1 in, 2 out]
                }
              }
            }
          }
        }
        n178 = call <vilib>:"Add State(s) to Queue__jki_lib_state_machine.vi"("State(s) in (\"\")"=w377) -> ("States Out"=w376:string)  [unwired: 14 in]
      }
      frame "UI: Cursor Set" {
        # "Argument"
        # "Set and Unset Cursor Busy.\n(Usage: \"UI: Cursor Set >> Busy|Idle\")"
        n179 = case shown="\"Busy\"" w385 {
          tunnel: w387 -> [w392 w394]
          tunnel: [w391 w393] -> w386
          frame "Idle", Default {
            n180 = call <vilib>:"Unset Busy.vi"("error in (no error)"=w392) -> ("error out"=w391:errorcluster)  [unwired: 10 in]
          }
          frame "Busy" {
            n181 = call <vilib>:"Set Busy.vi"("error in (no error)"=w394) -> ("error out"=w393:errorcluster)  [unwired: 9 in, 1 out]
          }
        }
        n182 = call <vilib>:"Add State(s) to Queue__jki_lib_state_machine.vi"("State(s) in (\"\")"=w390) -> ("States Out"=w389:string)  [unwired: 14 in]
      }
      frame "UI: Front Panel State" {
        # "Argument"
        # "Set Front Panel Open or Closed\n(Usage: \"UI: Front Panel State >> Open|Close\")"
        n183 = Unbundle By Name(w397) -> ("Core.Current VI Reference"=w396:refnum<vi>)
        n184 = case shown="\"Open\", \"Standard\", Default" w395 {
          tunnel: w399 -> [w407 w422 w433 w446 w459]
          tunnel: [w409 w423 w435 w448 w461] -> w398
          tunnel: w396 -> [w408 w420 w434 w447 w460]
          frame "Open", "Standard", Default {
            w402 = T2."Standard" ("State")
            n185 = property class="VI"(reference=w408, error in=w407) -> (reference out=w405:refnum<vi>, error out=w406:errorcluster, "FP.State"=w404:T2)
            n186 = Not Equal?(x=w404, y=w402) -> (x != y?=w403:bool)
            n187 = case shown="False" w403 {
              tunnel: [w413 w415] -> w409
              tunnel: w406 -> [w412 w415]
              tunnel: w405 -> [w411 _]
              tunnel: w402 -> [w410 _]
              frame True {
                n188 = invoke class="VI" method="FP.Open"(reference=w411, error in=w412, "Activate"=TRUE, "State"=w410) -> (error out=w413:errorcluster)  [unwired: 1 in, 4 out]
              }
              frame False {
              }
            }
          }
          frame "Close", "Closed" {
            n189 = property class="VI"(reference=w420, error in=w422) -> (reference out=w419:refnum<vi>, error out=w421:errorcluster, "FP.State"=w417:T2)
            n190 = Not Equal?(x=w417, y=T2."Closed" ("Front Panel Window:State")) -> (x != y?=w416:bool)
            n191 = case shown="True" w416 {
              tunnel: [w424 w427] -> w423
              tunnel: w421 -> [w424 w426]
              tunnel: w419 -> [_ w425]
              frame False {
              }
              frame True {
                n192 = invoke class="VI" method="FP.Close"(reference=w425, error in=w426) -> (error out=w427:errorcluster)  [unwired: 1 in, 2 out]
              }
            }
          }
          frame "Hidden", "Hide" {
            w428 = T2."Hidden" ("State")
            n193 = property class="VI"(reference=w434, error in=w433) -> (reference out=w431:refnum<vi>, error out=w432:errorcluster, "FP.State"=w430:T2)
            n194 = Not Equal?(x=w430, y=w428) -> (x != y?=w429:bool)
            n195 = case shown="True" w429 {
              tunnel: [w439 w440] -> w435
              tunnel: w432 -> [w438 w440]
              tunnel: w431 -> [w437 _]
              tunnel: w428 -> [w436 _]
              frame True {
                n196 = invoke class="VI" method="FP.Open"(reference=w437, error in=w438, "State"=w436) -> (error out=w439:errorcluster)  [unwired: 2 in, 4 out]
              }
              frame False {
              }
            }
          }
          frame "Minimize", "Minimized" {
            w441 = T2."Minimized" ("State")
            n197 = property class="VI"(reference=w447, error in=w446) -> (reference out=w444:refnum<vi>, error out=w445:errorcluster, "FP.State"=w443:T2)
            n198 = Not Equal?(x=w443, y=w441) -> (x != y?=w442:bool)
            n199 = case shown="True" w442 {
              tunnel: [w452 w453] -> w448
              tunnel: w445 -> [w451 w453]
              tunnel: w444 -> [w450 _]
              tunnel: w441 -> [w449 _]
              frame True {
                n200 = invoke class="VI" method="FP.Open"(reference=w450, error in=w451, "State"=w449) -> (error out=w452:errorcluster)  [unwired: 2 in, 4 out]
              }
              frame False {
              }
            }
          }
          frame "Maximize", "Maximized" {
            w454 = T2."Maximized" ("State")
            n201 = property class="VI"(reference=w460, error in=w459) -> (reference out=w457:refnum<vi>, error out=w458:errorcluster, "FP.State"=w456:T2)
            n202 = Not Equal?(x=w456, y=w454) -> (x != y?=w455:bool)
            n203 = case shown="True" w455 {
              tunnel: [w465 w466] -> w461
              tunnel: w458 -> [w464 w466]
              tunnel: w457 -> [w463 _]
              tunnel: w454 -> [w462 _]
              frame True {
                n204 = invoke class="VI" method="FP.Open"(reference=w463, error in=w464, "State"=w462) -> (error out=w465:errorcluster)  [unwired: 2 in, 4 out]
              }
              frame False {
              }
            }
          }
        }
        n205 = call <vilib>:"Add State(s) to Queue__jki_lib_state_machine.vi"("State(s) in (\"\")"=w401) -> ("States Out"=w400:string)  [unwired: 14 in]
      }
      frame "---------- Macro ----------" {
        # "Do not put any code in this frame.\n(It is a separator no-op. You can make a copy of this frame to create a new Macro frame)"
        n206 = call <vilib>:"Add State(s) to Queue__jki_lib_state_machine.vi"("State(s) in (\"\")"=w470) -> ("States Out"=w469:string)  [unwired: 14 in]
      }
      frame "Macro: Initialize" {
        w471 = "Data: Initialize\nInitialize Core Data\nUI: Initialize\nUI: Front Panel State >> Open\n\nMacro: Read File"  # Data: Initialize Initialize Core Data UI: Initialize UI: Front Panel State >> Open  Macro: Read File
        # "Initialization Macro\n(This is called once, when the VI starts)"
        n207 = call <vilib>:"Add State(s) to Queue__jki_lib_state_machine.vi"("State(s) in Front (\"\")"=w471, "State(s) in (\"\")"=w475) -> ("States Out"=w474:string)  [unwired: 13 in]
      }
      frame "Macro: Read File" {
        # "Initialization Macro\n(This is called once, when the VI starts)"
        n208 = call <vilib>:"Add State(s) to Queue__jki_lib_state_machine.vi"("State(s) in Front (\"\")"="UI: Cursor Set >> Busy\nUI: Disable Buttons\nData: Choose File List\nData: Read File List\nData: Update Listbox\nUI: Enable Buttons\nUI: Cursor Set >> Idle", "State(s) in (\"\")"=w480) -> ("States Out"=w479:string)  [unwired: 13 in]
      }
      frame "Macro: Exit" {
        # "Exit Macro\n(This is called once, when the VI exits)"
        n209 = Unbundle By Name(w487) -> ("Core.Close Panel on Exit?"=w486:bool)
        n210 = Select(t="UI: Front Panel State >> Close", s=w486, f="") -> (s? t:f=w483:string)
        n211 = call <vilib>:"Add State(s) to Queue__jki_lib_state_machine.vi"("State(s) in (\"\")"=w483, "State(s) at Back (\"\")"="Data: Cleanup\nExit") -> ("States Out"=w481:string)  [unwired: 13 in]
        n212 = call <vilib>:"Add State(s) to Queue__jki_lib_state_machine.vi"("State(s) in Front (\"\")"=w481, "State(s) in (\"\")"=w490) -> ("States Out"=w489:string)  [unwired: 13 in]
      }
      frame "---------- VIPM ----------" {
        # "Template Separator\n(You can make a copy of, or modify, this frame)"
        n213 = call <vilib>:"Add State(s) to Queue__jki_lib_state_machine.vi"("State(s) in (\"\")"=w494) -> ("States Out"=w493:string)  [unwired: 14 in]
      }
      frame "VIPM: Open File" {
        # "Your code here.\n(You can make a copy of, or modify, this frame)"
        n214 = Unbundle By Name(w505) -> ("selected path"=w495:path)
        n215 = Format Into String(format string="cmd /c explorer.exe \"%s\"", error in=w499, w495) -> (resulting string=w503:string, error out=w501:errorcluster)  [unwired: 1 in]
        n216 = Strip Path(path=w495) -> (name=w497:string)  [unwired: 1 out]
        n217 = call <vilib>:"System Exec.vi"("run minimized? (F)"=TRUE, "error in (no error)"=w501, "command line"=w503) -> ("error out"=w500:errorcluster)  [unwired: 5 in, 3 out]
        n218 = Format Into String(format string="Opening \"%s\"...", w497) -> (resulting string=w498:string)  [unwired: 2 in, 1 out]
        n219 = local write "Status"(w498) -> ()
        n220 = call <vilib>:"Add State(s) to Queue__jki_lib_state_machine.vi"("State(s) in (\"\")"=w507) -> ("States Out"=w506:string)  [unwired: 14 in]
      }
      frame "VIPM: Preview VIPB" {
        # "Your code here.\n(You can make a copy of, or modify, this frame)"
        n221 = Unbundle By Name(w518) -> ("vipb paths"=w514:path[], "selected path"=w516:path)
        n222 = local read "ALL"() -> (w512:bool)
        n223 = Build Array(w516) -> (w513:path[])
        n224 = Select(t=w514, s=w512, f=w513) -> (s? t:f=w515:path[])
        n225 = for {
          tunnel: w515 -> [w524] mode=indexing
          tunnel: [w527] -> w510
          tunnel: w517 -> [w526]
          tunnel: [w525] -> w511 mode=indexing
          n226 = Strip Path(path=w524) -> (name=w521:string)  [unwired: 1 out]
          n227 = Format Into String(format string="Reading \"%s\"...", w521) -> (resulting string=w523:string)  [unwired: 2 in, 1 out]
          n228 = call <vilib>:"Read VI Package Build Spec_vipm_api.vi"("error in (no error)"=w526, "Path to VIPB File"=w524) -> ("error out"=w527:errorcluster, "VI Package Build Spec Data"=w525:T8)  [unwired: 8 in]
          n229 = local write "Status"(w523) -> ()
        }
        n230 = call "Format Build Spec Summary.vi"("error in (no error)"=w510, "Build Spec [] in"=w511) -> ("error out"=w509:errorcluster, "VIPB Preview"=w508:string)  [unwired: 8 in]
        n231 = local write "Status"(w508) -> ()
        n232 = call <vilib>:"Add State(s) to Queue__jki_lib_state_machine.vi"("State(s) in (\"\")"=w520) -> ("States Out"=w519:string)  [unwired: 14 in]
      }
      frame "VIPM: Increment Patch" {
        # "Your code here.\n(You can make a copy of, or modify, this frame)"
        n233 = Unbundle By Name(w538) -> ("vipb paths"=w535:path[], "selected path"=w537:path)
        n234 = local read "ALL"() -> (w532:bool)
        n235 = Build Array(w537) -> (w534:path[])
        n236 = Select(t=w535, s=w532, f=w534) -> (s? t:f=w536:path[])
        n237 = for {
          tunnel: w536 -> [w542] mode=indexing
          tunnel: w533 -> [w547]
          tunnel: [w543] -> w531
          tunnel: [w541] -> w529 mode=indexing
          n238 = Strip Path(path=w542) -> (name=w544:string)  [unwired: 1 out]
          n239 = Format Into String(format string="Updating \"%s\"...", w544) -> (resulting string=w546:string)  [unwired: 2 in, 1 out]
          n240 = call "Increment Patch.vi"("error in (no error)"=w547, "selected path"=w542) -> ("error out"=w543:errorcluster, "VI Package Build Spec Data"=w541:T8)  [unwired: 8 in]
          n241 = local write "Status"(w546) -> ()
        }
        n242 = call "Format Build Spec Summary.vi"("error in (no error)"=w531, "Build Spec [] in"=w529) -> ("error out"=w530:errorcluster, "VIPB Preview"=w528:string)  [unwired: 8 in]
        n243 = local write "Status"(w528) -> ()
        n244 = call <vilib>:"Add State(s) to Queue__jki_lib_state_machine.vi"("State(s) in (\"\")"=w540) -> ("States Out"=w539:string)  [unwired: 14 in]
      }
      frame "VIPM: Clear Notes" {
        # "Your code here.\n(You can make a copy of, or modify, this frame)"
        n245 = Unbundle By Name(w558) -> ("vipb paths"=w555:path[], "selected path"=w557:path)
        n246 = local read "ALL"() -> (w552:bool)
        n247 = Build Array(w557) -> (w554:path[])
        n248 = Select(t=w555, s=w552, f=w554) -> (s? t:f=w556:path[])
        n249 = for {
          tunnel: w556 -> [w561] mode=indexing
          tunnel: w553 -> [w567]
          tunnel: [w562] -> w551 mode=indexing
          tunnel: [w563] -> w550
          n250 = Strip Path(path=w561) -> (name=w564:string)  [unwired: 1 out]
          n251 = Format Into String(format string="Updating \"%s\"...", w564) -> (resulting string=w566:string)  [unwired: 2 in, 1 out]
          n252 = call "Clear Change Log.vi"("error in (no error)"=w567, "selected path"=w561) -> ("error out"=w563:errorcluster, "VI Package Build Spec Data"=w562:T8)  [unwired: 8 in]
          n253 = local write "Status"(w566) -> ()
        }
        n254 = call "Format Build Spec Summary.vi"("error in (no error)"=w550, "Build Spec [] in"=w551) -> ("error out"=w549:errorcluster, "VIPB Preview"=w548:string)  [unwired: 8 in]
        n255 = local write "Status"(w548) -> ()
        n256 = call <vilib>:"Add State(s) to Queue__jki_lib_state_machine.vi"("State(s) in (\"\")"=w560) -> ("States Out"=w559:string)  [unwired: 14 in]
      }
      frame "VIPM: Append Notes" {
        # "Your code here.\n(You can make a copy of, or modify, this frame)"
        n257 = Unbundle By Name(w577) -> ("vipb paths"=w574:path[], "selected path"=w576:path)
        n258 = local read "ALL"() -> (w571:bool)
        n259 = Build Array(w576) -> (w573:path[])
        n260 = Select(t=w574, s=w571, f=w573) -> (s? t:f=w575:path[])
        n261 = for {
          tunnel: w575 -> [w580] mode=indexing
          tunnel: w572 -> [w587]
          tunnel: [w583] -> w570
          tunnel: [w582] -> w569 mode=indexing
          n262 = Strip Path(path=w580) -> (name=w584:string)  [unwired: 1 out]
          n263 = Format Into String(format string="Updating \"%s\"...", w584) -> (resulting string=w586:string)  [unwired: 2 in, 1 out]
          n264 = call "Append to Change Log.vi"("error in (no error)"=w587, "Release Notes"="Release Notes", "selected path"=w580) -> ("error out"=w583:errorcluster, "VI Package Build Spec Data"=w582:T8)  [unwired: 7 in]
          n265 = local write "Status"(w586) -> ()
        }
        n266 = call "Format Build Spec Summary.vi"("Build Spec [] in"=w569) -> ("VIPB Preview"=w568:string)  [unwired: 9 in, 1 out]
        n267 = local write "Status"(w568) -> ()
        n268 = call <vilib>:"Add State(s) to Queue__jki_lib_state_machine.vi"("State(s) in (\"\")"=w579) -> ("States Out"=w578:string)  [unwired: 14 in]
      }
      frame "VIPM: Build VIPB" {
        # "Template Separator\n(You can make a copy of, or modify, this frame)"
        n269 = Unbundle By Name(w595) -> ("vipb paths"=w600:path[], "selected path"=w602:path)
        n270 = local read "ALL"() -> (w590:bool)
        n271 = Build Array(w602) -> (w599:path[])
        n272 = Select(t=w600, s=w590, f=w599) -> (s? t:f=w601:path[])
        n273 = for {
          tunnel: w601 -> [w605] mode=indexing
          tunnel: [w611] -> w598
          tunnel: w597 -> [w610]
          tunnel: [w609] -> w594 mode=indexing
          n274 = Strip Path(path=w605) -> (name=w606:string)  [unwired: 1 out]
          n275 = Format Into String(format string="Building \"%s\"...", w606) -> (resulting string=w608:string)  [unwired: 2 in, 1 out]
          n276 = local write "Status"(w608) -> ()
          n277 = call <vilib>:"Build VI Package_vipm_api.vi"("error in (no error)"=w610, "Path to VIPB File"=w605) -> ("error out"=w611:errorcluster, "Build Output"=w609:path)  [unwired: 8 in]
        }
        n278 = call <vilib>:"Build State String with Arguments__JKI_lib_State_Machine.vi"("Arguments (\"\")"=w592, "State"="VIPM: Preview VIPB" ("State(s) in Front (\"\")")) -> ("State with Arguments"=w593:string)  [unwired: 4 in]
        n279 = Bundle By Name(cluster=w595, "vip paths"=w594) -> (w596:T5)
        n280 = property on="Mode" class="Enum (strict)"("Val(Sgnl)"=File_Type--enum."Package (vip)" ("Value (Signaling)")) -> ()  [unwired: 2 in, 2 out]
        n281 = call <vilib>:"Add State(s) to Queue__jki_lib_state_machine.vi"("State(s) in Front (\"\")"=w593, "State(s) in (\"\")"=w604, "State(s) at Back (\"\")"="Data: Update Listbox" ("State(s) at Back (\"\")")) -> ("States Out"=w603:string)  [unwired: 12 in]
      }
      frame "VIPM: Publish VIPB" {
        # "Template Separator\n(You can make a copy of, or modify, this frame)"
        n282 = Unbundle By Name(w619) -> ("vip paths"=w618:path[])
        n283 = call <vilib>:"List VIPM Managed Repositories_vipm_api.vi"("error in (no error)"=w616) -> ("Managed Repositories Info"=w620:T10[], "error out"=w621:errorcluster)  [unwired: 13 in]
        n284 = Index Array(array=w620) -> (element=w622:T10)  [unwired: 1 in]
        n285 = Unbundle By Name(w622) -> ("Repository Name"=w623:string)
        n286 = call <vilib>:"Publish VI Packages to Repository_vipm_api.vi"("error in (no error)"=w621, "Repository Name"=w623, "Packages to publish to Repository Library (vip,ogp)"=w618) -> ("error out"=w617:errorcluster, "Package Names Published"=w613:string[])  [unwired: 7 in]
        n287 = Build Array (concatenate)("Packages Published:", w613) -> (w612:string[])
        n288 = call <vilib>:"1D String Array to Delimited String.vi"("delimiter"="\n", "string array"=w612) -> ()  [unwired: 9 in, 1 out]
        n289 = call <vilib>:"Add State(s) to Queue__jki_lib_state_machine.vi"("State(s) in (\"\")"=w625) -> ("States Out"=w624:string)  [unwired: 14 in]
      }
    }
  }
